vi "TCP Get Request.vi"(8 "error in (no error)":errorcluster, 11 "TCP Network Connection in":refnum<k5>) -> (0 "error out":errorcluster, 2 "data out":string, 3 "TCP Network Connection out":refnum<k5>)   [LabVIEW 2015]
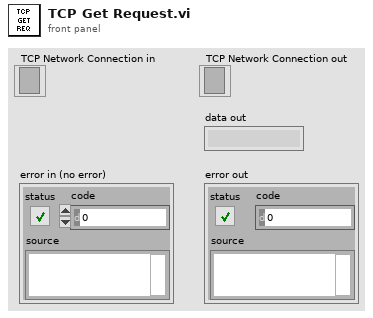
[diagram p1: front panel]
types:
  T1 = enum16{"Standard", "Buffered", "CRLF", "Immediate"}
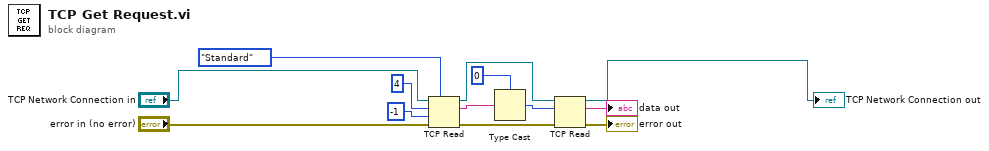
[diagram p0: block diagram]
diagram:
  n1 = TCP Read(connection ID="TCP Network Connection in", bytes to read=4, error in (no error)="error in (no error)", 7:T1."Standard" ("mode (standard)"), 9:-1 ("timeout ms (25000)")) -> (connection ID out=w8:refnum<k5>, data out=w5:string, error out=w10:errorcluster)
  n2 = Type Cast(type=0 ("bytes to read"), x=w5) -> (*(type *) &x=w7:i32)
  n3 = TCP Read(connection ID=w8, bytes to read=w7, error in (no error)=w10) -> (connection ID out=→"TCP Network Connection out":refnum<k5>, data out=→"data out":string, error out=→"error out":errorcluster)  [unwired: 2 in]
